vi "Temperature Scan.vi"() -> ()   [LabVIEW 2021]
panel:
  in  "Temp Chan":string="T8"
  in  "Final Temp K":dbl=0.026 format="%#_13g"
  out "error out":errorcluster
  in  "Start Book Number":i32=352
  in  "error in (no error)":errorcluster
  in  "Temperature List K":dbl[](array[numeric])=[0.05, 0.1, 0.15, 0.2, 0.25, 0.3, 0.4, 0.5, 0.6, 0.8, 1.0] format="%.3f"
  in  "DR  Address":string="mrl-dvh-triton.mrl.illinois.edu"
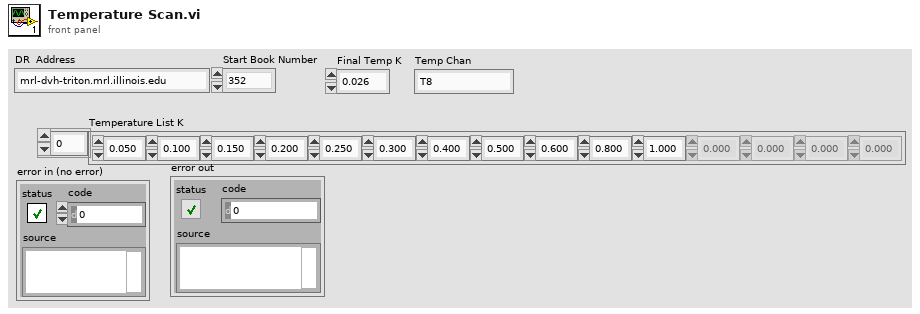
[diagram p1: front panel]
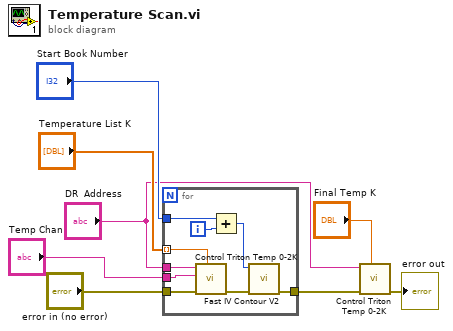
[diagram p0: block diagram]
diagram:
  n1 = for {
    tunnel: "Temperature List K" -> [w16] mode=indexing
    tunnel: "error in (no error)" -> [w17]
    tunnel: "Start Book Number" -> [w13]
    tunnel: [w11] -> w3
    tunnel: "DR  Address" -> [w10]
    tunnel: "Temp Chan" -> [w9]
    i -> [w14]
    n2 = call "Control Triton Temp 0-2K.vi"("Target Temperature K"=w16, "error in (no error)"=w17, "Temp Chan"=w9, "IP Address"=w10) -> ("error out"=w15:errorcluster)  [unwired: 7 in]
    n3 = Add(x=w13, y=w14) -> (x+y=w12:i32)
    n4 = call "Fast IV Contour V2.vi"("error in"=w15, "Book number"=w12) -> ("error out"=w11:errorcluster)  [unwired: 9 in]
  }
  n5 = call "Control Triton Temp 0-2K.vi"("Target Temperature K"="Final Temp K", "error in (no error)"=w3, "IP Address"="DR  Address") -> ("error out"=→"error out":errorcluster)  [unwired: 8 in]
